vi "Join strings by delimiter.vi"(7 "Delimiter":string, 10 "Strings []":string[](array[string]), 11 "Expand Symbols? (T)":bool=TRUE) -> (2 "String Out":string)   [LabVIEW 2015, in "Case Manipulation.lvlib"]
uses:
  Case Manipulation.lvlib
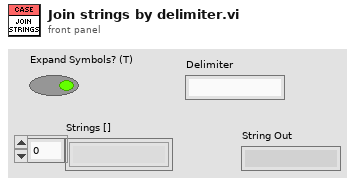
[diagram p1: front panel]
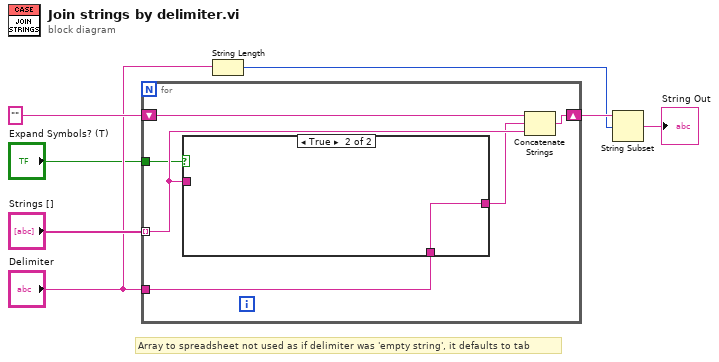
[diagram p0: block diagram]
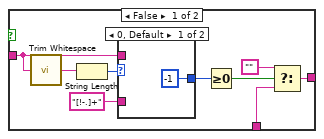
[diagram p2: hidden frame]
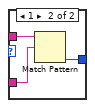
[diagram p3: hidden frame]
diagram:
  # "Array to spreadsheet not used as if delimiter was 'empty string', it defaults to tab"
  n1 = for {
    tunnel: "Strings []" -> [w11] mode=indexing
    tunnel: "Delimiter" -> [w10]
    shift-right: [w13] -> w5
    shift-left: "" -> [w12]
    tunnel: "Expand Symbols? (T)" -> [w8]
    n2 = case shown="True" w8 {
      tunnel: w11 -> [w21 _]
      tunnel: w10 -> [w17 w27]
      tunnel: [w16 w27] -> w9
      frame False {
        n3 = call <vilib>:"Trim Whitespace.vi"("string"=w21) -> ("trimmed string"=w14:string)  [unwired: 1 in]
        n4 = String Length(string=w14) -> (length=w22:i32)
        n5 = case shown="0, Default" w22 {
          tunnel: w21 -> [_ w26]
          tunnel: "[!-.]+" ("regular expression") -> [_ w25]
          tunnel: [-1 ("offset past match") w24] -> w19
          frame 0, Default {
          }
          frame 1 {
            n6 = Match Pattern(string=w26, regular expression=w25) -> (offset past match=w24:i32)  [unwired: 1 in, 3 out]
          }
        }
        n7 = Greater Or Equal To 0?(x=w19) -> (x >= 0?=w18:bool)
        n8 = Select(t="", s=w18, f=w17) -> (s? t:f=w16:string)
      }
      frame True {
      }
    }
    n9 = Concatenate Strings(w12, w9, w11) -> (w13:string)
  }
  n10 = String Length(string="Delimiter") -> (length=w3:i32)
  n11 = String Subset(string=w5, offset (0)=w3) -> (substring=→"String Out":string)  [unwired: 1 in]
